vi "Hologram.vi"() -> ()   [LabVIEW 2015]
uses:
  <vilib>/Math Plots/3D Math Plots/3D Surface/3D Surface XCtrl/3D Surface.xctl
  <vilib>/Analysis/2dsp.llb/2D Real FFT.vi
  <vilib>/Analysis/2dsp.llb/2D Inverse Complex FFT.vi
  <vilib>/Math Plots/3D Math Plots/3D Surface/3D Surface Datatype/Public/Plot Helper (Matrix).vi
  <vilib>/gmath/interp.llb/Create Mesh Grid (2D) (x,y arrays).vi
  <vilib>/Math Plots/3D Math Plots/3D Surface/3D Surface Datatype/3D Surface Datatype.lvclass
  <vilib>/gmath/NI_Gmath.lvlib
  <vilib>/Analysis/NI_AALPro.lvlib
panel:
  out "Array 5":dbl[](array[numeric])
  out "Array 4":dbl[](array[numeric])
  out "Array 3":dbl[][](array[numeric])
  out "angle(ifft)":picture
  out "abs ifft":refnum<class "3D Plot Datatype.lvclass">[](xcontrol)
  out "ifft of Mask":picture
  out "Array 2":cdb[][](array[numeric])
  out "Array":dbl[][](array[numeric])
  out "Mask":picture
  out "log Fih":dbl[][](array[numeric])
  out "pt 2":cdb[][](array[numeric]) format="%#_1g"
  out "KX  + KY":cdb[][](array[numeric])
  out "KY":dbl[][](array[numeric])
  out "KX":dbl[][](array[numeric])
  out "ref wave raw":cdb[][](array[numeric]) format="%#_2g"
  out "Numeric 5":cdb
  out "Numeric 4":cdb
  out "Numeric 3":dbl
  out "Numeric 2":cdb
  out "Phi exp":cdb[][](array[numeric])
  out "Phi":cdb[][](array[numeric])
  out "Oringinal Image 2":dbl[][](array[numeric])
  out "Hologram":dbl[][](array[numeric])
  out "ref wave u8":dbl[][](array[numeric])
  out "IH":dbl[][](array[numeric])
  out "255*H/max":dbl[][](array[numeric])
  out "H/max":dbl[][](array[numeric])
  out "Max value":dbl format="%#_5g"
  out "Objwave":dbl[][](array[numeric])
  out "Oringinal Image":dbl[][](array[numeric])
  out "Fourier Space":picture
  out "Fih":picture
  out "FIH":dbl[][](array[numeric])
  out "Hologram":picture
  out "Reference Wave":picture
  out "Object Wave":picture
  out "Original Image 2":refnum<class "3D Plot Datatype.lvclass">[](xcontrol)
  in  "Path":path
  out "Original Image":refnum<class "3D Plot Datatype.lvclass">[](xcontrol)
  # "FIh"
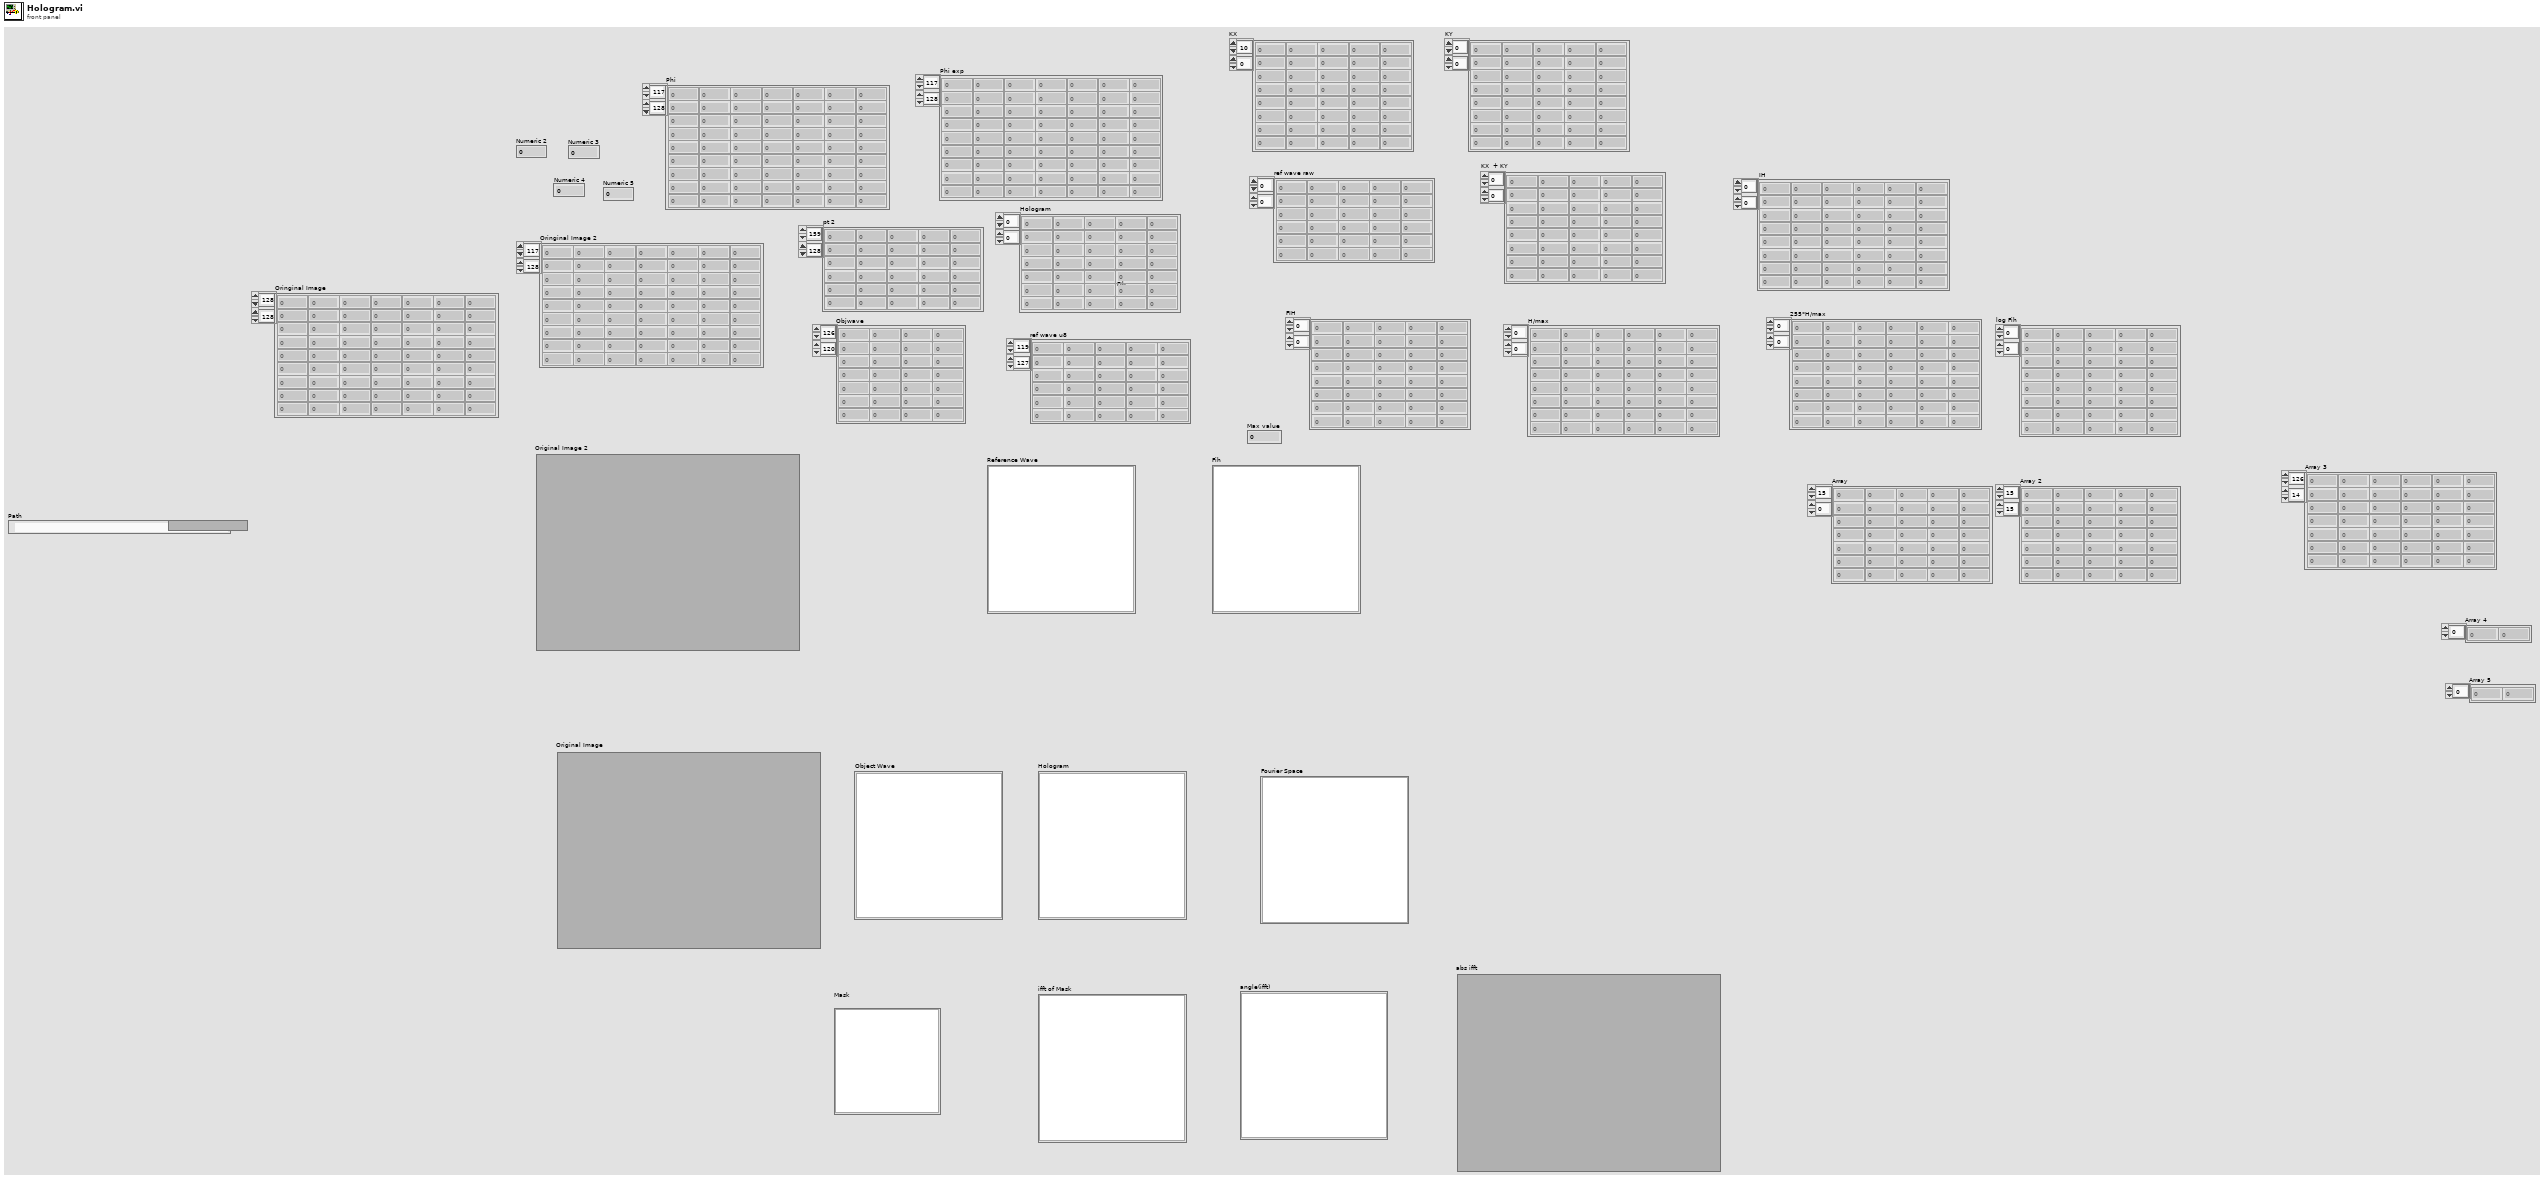
[diagram p1: front panel]
types:
  T1 = typedef "imagedata.ctl" = cluster{"image type":i32, "image depth":i32, "image":u8[], "mask":u8[], "colors":u32[], "Rectangle":cluster{"left":i16, "top":i16, "right":i16, "bottom":i16}}
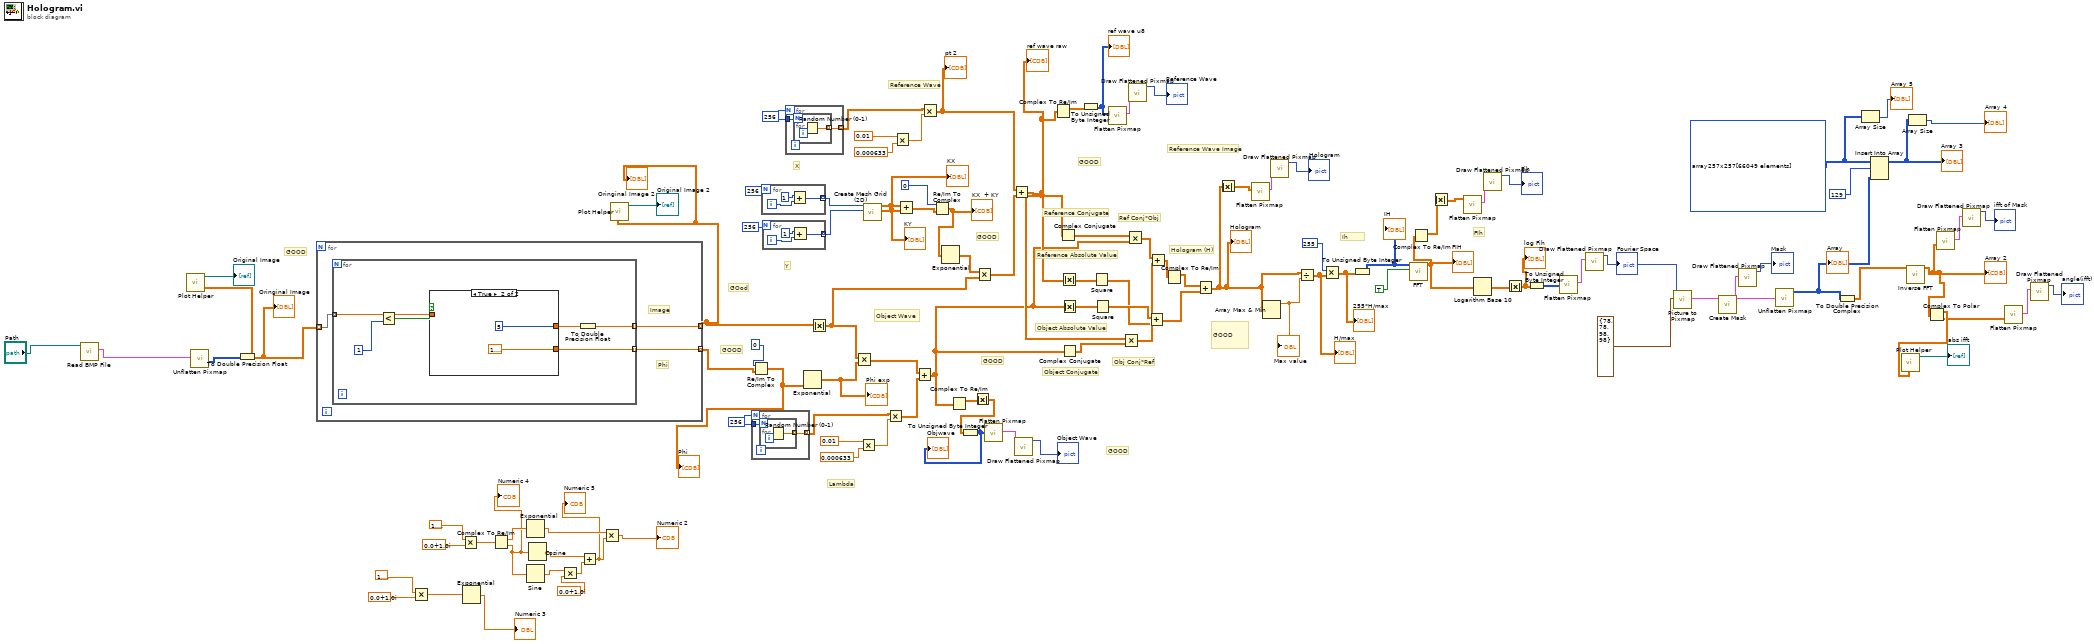
[diagram p0: block diagram]
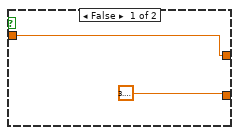
[diagram p2: hidden frame]
diagram:
  w2 = i32[][] array257x257[66049 elements]
  w98 = 256
  w111 = 256
  # "GOOD"
  # "GOOD"
  # "GOOD"
  # "GOOD"
  # "GOOD"
  # "GOOD"
  # "GOod"
  # "GOOD"
  # "FIh"
  # "Ih"
  # "Hologram (H)"
  # "Ref Conj*Obj"
  # "Obj Conj*Ref"
  # "Reference Conjugate"
  # "Reference Absolute Value"
  # "Object Absolute Value"
  # "Object Conjugate"
  # "Reference Wave Image"
  # "Y"
  # "X"
  # "Lambda"
  # "Reference Wave"
  # "Object Wave"
  n1 = call <vilib>:"Read BMP File.vi"("path to BMP file"="Path") -> ("image data"=w72:T1)  [unwired: 8 in, 2 out]
  n2 = call <vilib>:"Unflatten Pixmap.vi"("image data"=w72) -> ("4-bit pixmap"=w18:u8[][])  [unwired: 4 in, 6 out]
  n3 = To Double Precision Float(number=w18) -> (double precision float=w70:dbl[][])
  "Oringinal Image" <- w70
  n4 = call-poly <vilib>:"Plot Helper.vi"("z matrix"=w70) -> ("3D Plot lvclass Array out"=→"Original Image":refnum<class "3D Plot Datatype.lvclass">[])  [unwired: 5 in, 5 out]
  n5 = for {
    tunnel: w70 -> [w116] mode=indexing
    tunnel: [w115] -> w66 mode=indexing
    tunnel: [w114] -> w48 mode=indexing
    # "Phi"
    # "Image"
    n6 = for {
      tunnel: w116 -> [w117] mode=indexing
      tunnel: [w121] -> w115 mode=indexing
      tunnel: [w118] -> w114 mode=indexing
      n7 = Less?(x=w117, y=1) -> (x < y?=w120:bool)
      n8 = case shown="True" w120 {
        tunnel: [w123 5] -> w122
        tunnel: [3.141592653589793 1.5707963267948966] -> w118
        tunnel: w117 -> [w123 _]
        frame False {
        }
        frame True {
        }
      }
      n9 = To Double Precision Float(number=w122) -> (double precision float=w121:dbl)
    }
  }
  "Oringinal Image 2" <- w66
  n10 = Multiply(x=1.5707963267948966, y=cdb 0.0+1.0i) -> (x*y=w61:cdb)
  n11 = Multiply(x=1.5707963267948966, y=cdb 0.0+1.0i) -> (x*y=w54:cdb)
  n12 = Exponential(1:w61) -> (0:→"Numeric 3":cdb)
  n13 = Complex To Re/Im(x + iy=w54) -> (x=w59:dbl, y=w52:dbl)
  "Numeric 4" <- w52
  n14 = Exponential(1:w59) -> (0:w53:dbl)
  n15 = Sine(x=w52) -> (sin(x)=w49:dbl)
  n16 = Cosine(x=w52) -> (cos(x)=w50:dbl)
  n17 = Multiply(x=w49, y=cdb 0.0+1.0i) -> (x*y=w57:cdb)
  n18 = Add(x=w50, y=w57) -> (x+y=w51:cdb)
  "Numeric 5" <- w51
  n19 = Multiply(x=w53, y=w51) -> (x*y=→"Numeric 2":cdb)
  n20 = call-poly <vilib>:"Plot Helper.vi"("z matrix"=w66) -> ("3D Plot lvclass Array out"=→"Original Image 2":refnum<class "3D Plot Datatype.lvclass">[])  [unwired: 5 in, 5 out]
  n21 = for {
    N: w111 -> [_]
    tunnel: w111 -> [w128]
    tunnel: [w127] -> w108 mode=indexing
    n22 = for {
      N: w128 -> [_]
      tunnel: [w129] -> w127 mode=indexing
      n23 = Random Number (0-1)() -> (number: 0 to 1=w129:dbl)
    }
  }
  n24 = Re/Im To Complex(1:w48, 2:0) -> (0:w47:cdb[][])
  "Phi" <- w47
  n25 = for {
    N: 256 -> [_]
    tunnel: [w130] -> w91 mode=indexing
    i -> [w131]
    n26 = Add(x=1, y=w131) -> (x+y=w130:i32)
  }
  n27 = for {
    N: 256 -> [_]
    tunnel: [w133] -> w100 mode=indexing
    i -> [w134]
    n28 = Add(x=1, y=w134) -> (x+y=w133:i32)
  }
  n29 = for {
    N: w98 -> [_]
    tunnel: w98 -> [w137]
    tunnel: [w136] -> w92 mode=indexing
    n30 = for {
      N: w137 -> [_]
      tunnel: [w138] -> w136 mode=indexing
      n31 = Random Number (0-1)() -> (number: 0 to 1=w138:dbl)
    }
  }
  n32 = Exponential(1:w47) -> (0:w65:cdb[][])
  "Phi exp" <- w65
  n33 = Absolute Value(x=w66) -> (abs(x)=w99:dbl[][])
  n34 = Multiply(x=w99, y=w65) -> (x*y=w106:cdb[][])
  n35 = Multiply(x=0.01, y=0.000633) -> (x*y=w107:dbl)
  n36 = call-poly <vilib>:"Create Mesh Grid (2D).vi"("y domain"=w100, "x domain"=w91) -> ("Y"=w44:dbl[][], "X"=w45:dbl[][])  [unwired: 7 in, 1 out]
  "KX" <- w45
  "KY" <- w44
  n37 = Multiply(x=w108, y=w107) -> (x*y=w105:dbl[][])
  n38 = Multiply(x=0.01, y=0.000633) -> (x*y=w95:dbl)
  n39 = Add(x=w45, y=w44) -> (x+y=w42:dbl[][])
  n40 = Add(x=w106, y=w105) -> (x+y=w34:cdb[][])
  n41 = Multiply(x=w92, y=w95) -> (x*y=w38:dbl[][])
  "pt 2" <- w38
  n42 = Re/Im To Complex(1:w42, 2:0) -> (0:w41:cdb[][])
  "KX  + KY" <- w41
  n43 = Exponential(1:w41) -> (0:w40:cdb[][])
  n44 = Complex To Re/Im(x + iy=w34) -> (x=w69:dbl[][])  [unwired: 1 out]
  n45 = Absolute Value(x=w69) -> (abs(x)=w26:dbl[][])
  n46 = To Unsigned Byte Integer(number=w26) -> (unsigned 8bit integer=w25:u8[][])
  "Objwave" <- w25
  n47 = Multiply(x=w40, y=w99) -> (x*y=w39:cdb[][])
  n48 = call <vilib>:"Flatten Pixmap.vi"("8-bit pixmap"=w25) -> ("image data"=w104:T1)  [unwired: 10 in]
  n49 = Add(x=w38, y=w39) -> (x+y=w36:cdb[][])
  "ref wave raw" <- w36
  n50 = call <vilib>:"Draw Flattened Pixmap.vi"("image data"=w104) -> ("new picture"=→"Object Wave":picture)  [unwired: 8 in]
  n51 = Complex To Re/Im(x + iy=w36) -> (x=w37:dbl[][])  [unwired: 1 out]
  n52 = Complex Conjugate(1:w36) -> (0:w73:cdb[][])
  n53 = Absolute Value(x=w36) -> (abs(x)=w89:dbl[][])
  n54 = Absolute Value(x=w34) -> (abs(x)=w90:dbl[][])
  n55 = Complex Conjugate(1:w34) -> (0:w88:cdb[][])
  n56 = To Unsigned Byte Integer(number=w37) -> (unsigned 8bit integer=w35:u8[][])
  "ref wave u8" <- w35
  n57 = Square(x=w89) -> (x^2=w84:dbl[][])
  n58 = Square(x=w90) -> (x^2=w87:dbl[][])
  n59 = call <vilib>:"Flatten Pixmap.vi"("8-bit pixmap"=w35) -> ("image data"=w94:T1)  [unwired: 10 in]
  n60 = Multiply(x=w36, y=w88) -> (x*y=w85:cdb[][])
  n61 = Multiply(x=w73, y=w34) -> (x*y=w86:cdb[][])
  n62 = call <vilib>:"Draw Flattened Pixmap.vi"("image data"=w94) -> ("new picture"=→"Reference Wave":picture)  [unwired: 8 in]
  n63 = Add(x=w87, y=w84) -> (x+y=w76:dbl[][])
  n64 = Add(x=w86, y=w85) -> (x+y=w75:cdb[][])
  n65 = Complex To Re/Im(x + iy=w75) -> (x=w74:dbl[][])  [unwired: 1 out]
  n66 = Add(x=w74, y=w76) -> (x+y=w33:dbl[][])
  "Hologram" <- w33
  n67 = Absolute Value(x=w33) -> (abs(x)=w27:dbl[][])
  n68 = call <vilib>:"Flatten Pixmap.vi"("8-bit pixmap"=w27) -> ("image data"=w82:T1)  [unwired: 10 in]
  n69 = Array Max & Min(array=w33) -> (max value=w32:dbl)  [unwired: 3 out]
  "Max value" <- w32
  n70 = call <vilib>:"Draw Flattened Pixmap.vi"("image data"=w82) -> ("new picture"=→"Hologram":picture)  [unwired: 8 in]
  n71 = Divide(x=w33, y=w32) -> (x/y=w68:dbl[][])
  "H/max" <- w68
  n72 = Multiply(x=255, y=w68) -> (x*y=w67:dbl[][])
  "255*H/max" <- w67
  n73 = To Unsigned Byte Integer(number=w67) -> (unsigned 8bit integer=w31:u8[][])
  "IH" <- w31
  n74 = call-poly <vilib>:"FFT.vi"("shift?"=TRUE, "X"=w31) -> ("FFT {X}"=w30:cdb[][])  [unwired: 8 in, 1 out]
  "FIH" <- w30
  n75 = Complex To Re/Im(x + iy=w30) -> (x=w78:dbl[][])  [unwired: 1 out]
  n76 = Absolute Value(x=w78) -> (abs(x)=w77:dbl[][])
  n77 = call <vilib>:"Flatten Pixmap.vi"("24-bit pixmap"=w77) -> ("image data"=w80:T1)  [unwired: 10 in]
  n78 = Logarithm Base 10(1:w30) -> (0:w29:cdb[][])
  n79 = call <vilib>:"Draw Flattened Pixmap.vi"("image data"=w80) -> ("new picture"=→"Fih":picture)  [unwired: 8 in]
  n80 = Absolute Value(x=w29) -> (abs(x)=w24:dbl[][])
  "log Fih" <- w24
  n81 = To Unsigned Byte Integer(number=w24) -> (unsigned 8bit integer=w28:u8[][])
  n82 = call <vilib>:"Flatten Pixmap.vi"("4-bit pixmap"=w28) -> ("image data"=w23:T1)  [unwired: 10 in]
  n83 = call <vilib>:"Draw Flattened Pixmap.vi"("image data"=w23) -> ("new picture"=w19:picture)  [unwired: 8 in]
  "Fourier Space" <- w19
  n84 = call <vilib>:"Picture to Pixmap.vi"("rect"=cluster{i16, i16, i16, i16} {78, 78, 98, 98}, "picture"=w19) -> ("image data"=w22:T1)  [unwired: 8 in, 1 out]
  n85 = call <vilib>:"Create Mask.vi"("image data"=w22) -> ("image data"=w17:T1)  [unwired: 10 in]
  n86 = call <vilib>:"Draw Flattened Pixmap.vi"("image data"=w17) -> ("new picture"=→"Mask":picture)  [unwired: 8 in]
  n87 = call <vilib>:"Unflatten Pixmap.vi"("image data"=w17) -> ("24-bit pixmap"=w6:u32[][])  [unwired: 4 in, 6 out]
  "Array" <- w6
  n88 = To Double Precision Complex(1:w6) -> (0:w15:cdb[][])
  n89 = Array Size(array=w2) -> (size(s)=→"Array 5":i32[])
  n90 = Insert Into Array(array=w2, index (row)=129, new element=w6) -> (w4:i32[][])  [unwired: 1 in]
  "Array 3" <- w4
  n91 = call-poly <vilib>:"Inverse FFT.vi"("FFT {x}"=w15) -> ("X"=w11:cdb[][])  [unwired: 9 in, 1 out]
  "Array 2" <- w11
  n92 = Array Size(array=w4) -> (size(s)=→"Array 4":i32[])
  n93 = Complex To Polar(r * e^(i*theta)=w11) -> (r=w10:dbl[][], theta=w7:dbl[][])
  n94 = call-poly <vilib>:"Plot Helper.vi"("z matrix"=w10) -> ("3D Plot lvclass Array out"=→"abs ifft":refnum<class "3D Plot Datatype.lvclass">[])  [unwired: 5 in, 5 out]
  n95 = call <vilib>:"Flatten Pixmap.vi"("4-bit pixmap"=w11) -> ("image data"=w14:T1)  [unwired: 10 in]
  n96 = call <vilib>:"Draw Flattened Pixmap.vi"("image data"=w14) -> ("new picture"=→"ifft of Mask":picture)  [unwired: 8 in]
  n97 = call <vilib>:"Flatten Pixmap.vi"("4-bit pixmap"=w7) -> ("image data"=w9:T1)  [unwired: 10 in]
  n98 = call <vilib>:"Draw Flattened Pixmap.vi"("image data"=w9) -> ("new picture"=→"angle(ifft)":picture)  [unwired: 8 in]
